vi "Set measurement.vi"(8 "error in (no error)":errorcluster, 10 "Measurement settings":T1={"Source Mode "=0, "Source Level"=0.01, "Source Limit"=0.01, "Remote sense"=TRUE, "Clear buffer?"=FALSE, "Beep"=TRUE, "High Capacity"=TRUE, "Terminals"=1, "PLCs"=2.0, "Fast measurement"=FALSE, "Measure Function"=2} {"Measure Function" items=["Volts", "Current", "Resistance"]; "Source Mode" items=["Voltage", "Current"]; "Terminals" items=["Front", "Rear"]}, 11 "VISA resource name":refnum<visa-resource-name>) -> (0 "error out":errorcluster, 1 "Measure Function":u16(ring)=2 items=["Volts", "Current", "Auto Resistance", "Manual Resistance", "Digitize Voltage", "Digitize Current"], 2 "Value":dbl, 3 "VISA resource name out":refnum<visa-resource-name>, 5 "Source Mode":u16(ring) items=["Voltage", "Current"])   [LabVIEW 2021]
uses:
  controls/SMU settings.ctl
  <instrlib>/Keithley 2450/Keithley 2450.lvlib
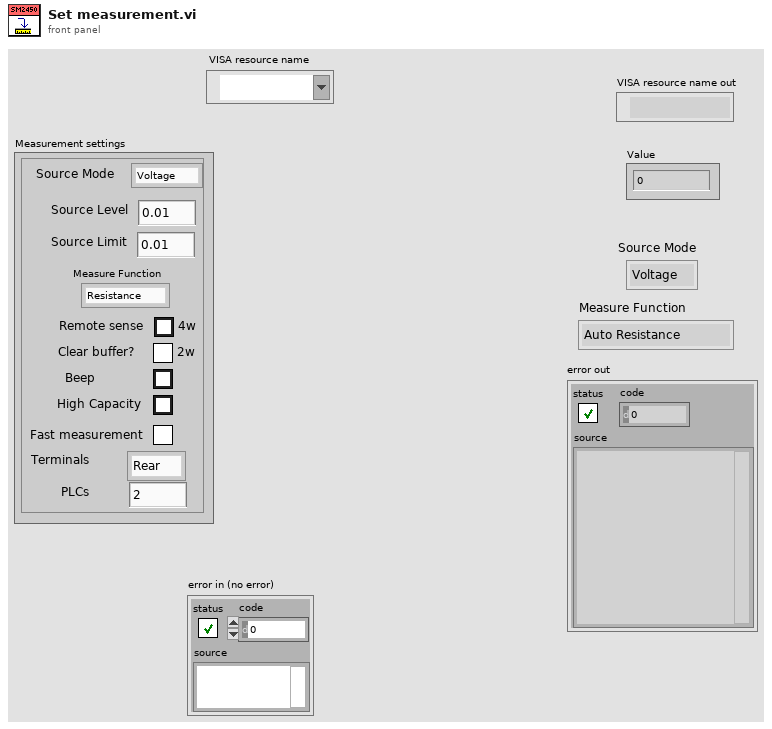
[diagram p1: front panel]
types:
  T1 = typedef "SMU settings.ctl" = cluster{"Source Mode ":u16, "Source Level":dbl, "Source Limit":dbl, "Remote sense":bool, "Clear buffer?":bool, "Beep":bool, "High Capacity":bool, "Terminals":u16, "PLCs":dbl, "Fast measurement":bool, "Measure Function":u16}
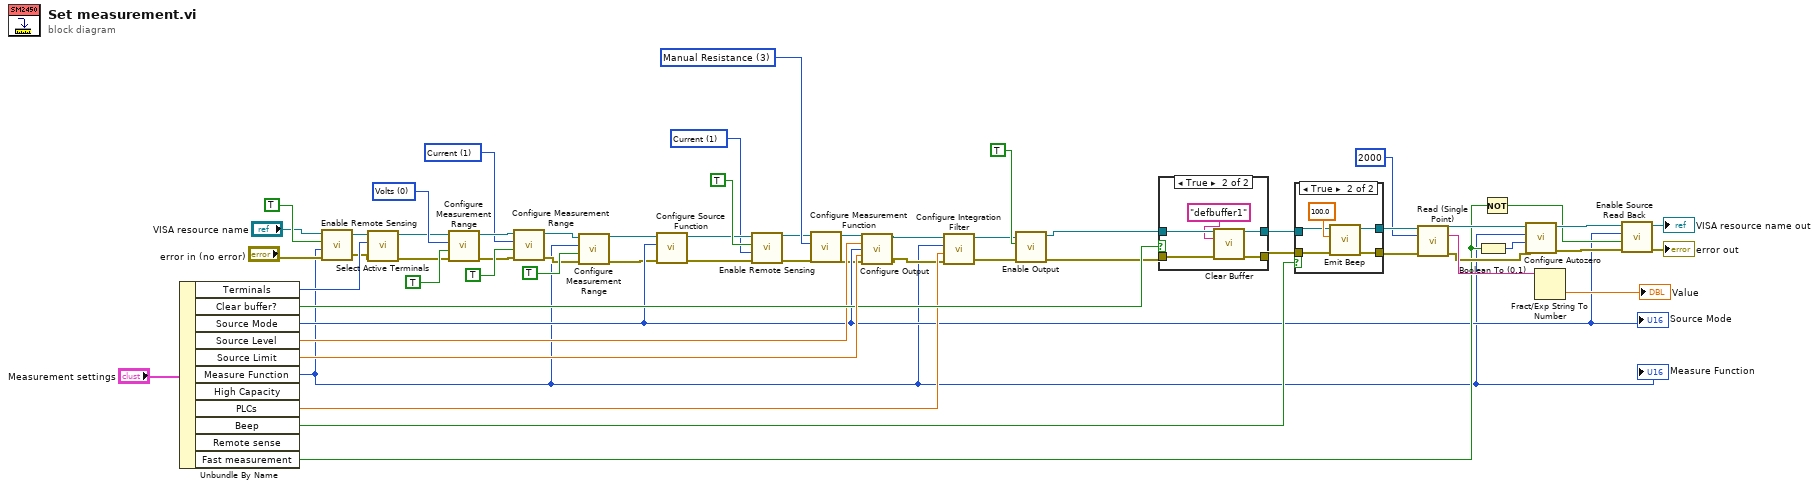
[diagram p0: block diagram]
diagram:
  w1 = u16 1 items=["Voltage", "Current", "Resistance", "Digitize Voltage", "Digitize Current"] ("Function (0:Voltage)")
  w15 = u16 3 items=["Volts", "Current", "Auto Resistance", "Manual Resistance", "Digitize Voltage", "Digitize Current"] ("Function (0: Volts)")
  w28 = u16 1 items=["Volts", "Current", "Resistance"] ("Function (0: Volts)")
  w29 = u16 0 items=["Volts", "Current", "Resistance"] ("Function (0: Volts)")
  n1 = Unbundle By Name("Measurement settings") -> ("Terminals"=w57:u16, "Clear buffer?"=w55:bool, "Source Mode"=w35:u16, "Source Level"=w45:dbl, "Source Limit"=w56:dbl, "Measure Function"=w2:u16, "PLCs"=w54:dbl, "Beep"=w51:bool, "Fast measurement"=w39:bool)  [unwired: 2 out]
  "Source Mode" <- w35
  "Measure Function" <- w2
  n2 = call <instrlib>:"Enable Remote Sensing.vi"("error in (no error)"="error in (no error)", "Function (0:Voltage)"=w2, "Enable Remote Sensing (T: Enable)"=TRUE, "VISA resource name"="VISA resource name") -> ("error out"=w5:errorcluster, "VISA resource name out"=w6:refnum<visa-resource-name>)  [unwired: 6 in]
  n3 = call <instrlib>:"Select Active Terminals.vi"("error in (no error)"=w5, "Active Terminals (0: Front)"=w57, "VISA resource name"=w6) -> ("error out"=w4:errorcluster, "VISA resource name out"=w3:refnum<visa-resource-name>)  [unwired: 7 in]
  n4 = call <instrlib>:"Configure Measurement Range.vi"("error in (no error)"=w4, "Enable Auto Range (T:Enable)"=TRUE, "Function (0: Volts)"=w29, "VISA resource name"=w3) -> ("error out"=w31:errorcluster, "VISA resource name out"=w30:refnum<visa-resource-name>)  [unwired: 6 in]
  n5 = call <instrlib>:"Configure Measurement Range.vi"("error in (no error)"=w31, "Enable Auto Range (T:Enable)"=TRUE, "Function (0: Volts)"=w28, "VISA resource name"=w30) -> ("error out"=w26:errorcluster, "VISA resource name out"=w27:refnum<visa-resource-name>)  [unwired: 6 in]
  n6 = call <instrlib>:"Configure Measurement Range.vi"("error in (no error)"=w26, "Enable Auto Range (T:Enable)"=TRUE, "Function (0: Volts)"=w2, "VISA resource name"=w27) -> ("error out"=w18:errorcluster, "VISA resource name out"=w19:refnum<visa-resource-name>)  [unwired: 6 in]
  n7 = call <instrlib>:"Configure Source Function.vi"("error in (no error)"=w18, "Function (0: Volts)"=w35, "VISA resource name"=w19) -> ("error out"=w13:errorcluster, "VISA resource name out"=w14:refnum<visa-resource-name>)  [unwired: 7 in]
  n8 = call <instrlib>:"Enable Remote Sensing.vi"("error in (no error)"=w13, "Function (0:Voltage)"=w1, "Enable Remote Sensing (T: Enable)"=TRUE, "VISA resource name"=w14) -> ("error out"=w12:errorcluster, "VISA resource name out"=w11:refnum<visa-resource-name>)  [unwired: 6 in]
  n9 = call <instrlib>:"Configure Measurement Function.vi"("error in (no error)"=w12, "Function (0: Volts)"=w15, "VISA resource name"=w11) -> ("error out"=w9:errorcluster, "VISA resource name out"=w10:refnum<visa-resource-name>)  [unwired: 7 in]
  n10 = call <instrlib>:"Configure Output.vi"("VISA resource name"=w10, "Source Level (0)"=w45, "Source Mode  (0: Voltage)"=w35, "Source Limit Level (0.1)"=w56, "error in (no error)"=w9) -> ("VISA resource name out"=w16:refnum<visa-resource-name>, "error out"=w17:errorcluster)  [unwired: 9 in]
  n11 = call <instrlib>:"Configure Integration Filter.vi"("error in (no error)"=w17, "Measurement Speed (1 PLC)"=w54, "Function (0: Volts)"=w2, "VISA resource name"=w16) -> ("error out"=w7:errorcluster, "VISA resource name out"=w8:refnum<visa-resource-name>)  [unwired: 6 in]
  n12 = call <instrlib>:"Enable Output.vi"("error in (no error)"=w7, "Enable Output (T: Enable)"=TRUE ("Enable Remote Sensing (T: Enable)"), "VISA resource name"=w8) -> ("error out"=w20:errorcluster, "VISA resource name out"=w21:refnum<visa-resource-name>)  [unwired: 7 in]
  n13 = case shown="True" w55 {
    tunnel: [w61 w66] -> w53
    tunnel: [w60 w65] -> w52
    tunnel: w20 -> [w61 w64]
    tunnel: w21 -> [w60 w63]
    frame False {
    }
    frame True {
      n14 = call <instrlib>:"Clear Buffer.vi"("VISA resource name"=w63, "Buffer Name (defbuffer1)"="defbuffer1", "error in (no error)"=w64) -> ("VISA resource name out"=w65:refnum<visa-resource-name>, "error out"=w66:errorcluster)  [unwired: 11 in]
    }
  }
  n15 = case shown="True" w51 {
    tunnel: [w67 w73] -> w49
    tunnel: [w68 w72] -> w50
    tunnel: w53 -> [w67 w70]
    tunnel: w52 -> [w68 w69]
    frame False {
    }
    frame True {
      n16 = call <instrlib>:"Emit Beep.vi"("error in (no error)"=w70, "Beep Frequency (300)"=100.0, "VISA resource name"=w69) -> ("error out"=w73:errorcluster, "VISA resource name out"=w72:refnum<visa-resource-name>)  [unwired: 7 in]
    }
  }
  n17 = call <instrlib>:"Read (Single Point).vi"("VISA resource name"=w50, "Timeout (10000 ms)"=2000, "error in (no error)"=w49) -> ("VISA resource name out"=w43:refnum<visa-resource-name>, "Data out"=w47:string, "error out"=w42:errorcluster)  [unwired: 10 in]
  n18 = Boolean To (0,1)(Boolean=w39) -> (0, 1=w44:i16)
  n19 = Not(x=w39) -> (.not. x?=w38:bool)
  n20 = call <instrlib>:"Configure Autozero.vi"("error in (no error)"=w42, "Autozero  (0: On)"=w44, "Function (0: Volts)"=w2, "VISA resource name"=w43) -> ("error out"=w40:errorcluster, "VISA resource name out"=w41:refnum<visa-resource-name>)  [unwired: 6 in]
  n21 = Fract/Exp String To Number(string=w47) -> (number=→"Value":dbl)  [unwired: 3 in, 1 out]
  n22 = call <instrlib>:"Enable Source Read Back.vi"("error in (no error)"=w40, "Enable Read Back  (T:Enable)"=w38, "Function (0: Volts)"=w35, "VISA resource name"=w41) -> ("error out"=→"error out":errorcluster, "VISA resource name out"=→"VISA resource name out":refnum<visa-resource-name>)  [unwired: 6 in]
